vi "GUI_CH1_Comm_ZEROMQ.vi"() -> ()   [LabVIEW 2018]
uses:
  RxTx/RxTx.lvclass
  <vilib>/addons/zeromq/socket_type.ctl
  <vilib>/addons/zeromq/zmq_context.lvclass
  <vilib>/addons/zeromq/zeromq.lvlib
  <vilib>/addons/zeromq/zmq_socket.lvclass
panel:
  out "error out 4":errorcluster
  out "error out":errorcluster
  in  "IP":string="200.131.64.49"
  in  "stop":bool
  out "error out 3":errorcluster
  out "error out 2":errorcluster
  in  "RxTx.lvclass 2":refnum<class "RxTx.lvclass">
  in  "Channel":u16=1
  # "Channel 1 - TCPIP Communication"
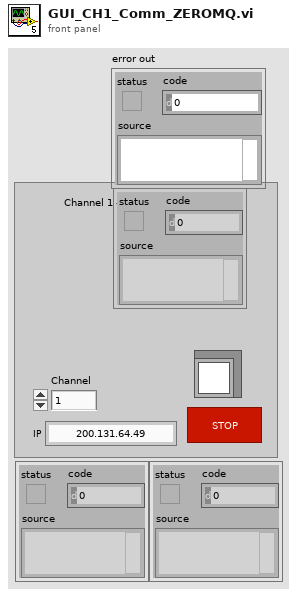
[diagram p1: front panel]
types:
  T1 = typedef "zeromq.lvlib/socket_type.ctl" = enum8{"ZMQ_PAIR", "ZMQ_PUB", "ZMQ_SUB", "ZMQ_REQ", "ZMQ_REP", "ZMQ_DEALER", "ZMQ_ROUTER", "ZMQ_PULL", "ZMQ_PUSH", "ZMQ_XPUB", "ZMQ_XSUB", "ZMQ_STREAM", "ZMQ_SERVER", "ZMQ_CLIENT", "ZMQ_RADIO", "ZMQ_DISH", "ZMQ_GATHER", "ZMQ_SCATTER", "ZMQ_DGRAM"}
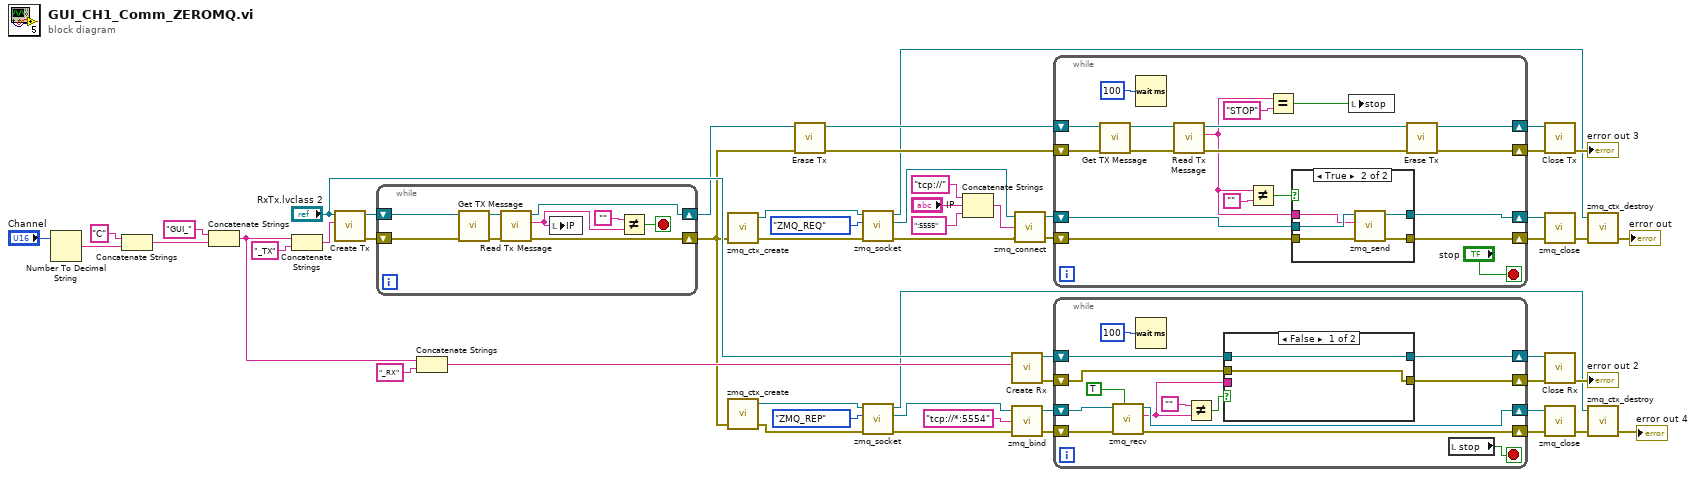
[diagram p0: block diagram]
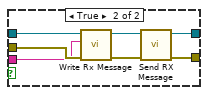
[diagram p3: hidden frame]
diagram:
  n1 = Number To Decimal String(number="Channel") -> (decimal integer string=w51:string)  [unwired: 1 in]
  n2 = Concatenate Strings("C", w51) -> (w36:string)
  n3 = Concatenate Strings("GUI_", w36) -> (w37:string)
  n4 = Concatenate Strings(w37, "_TX" ("Reader Name")) -> (w45:string)
  n5 = call "Create Tx.vi"("Writer Name"=w45, "RxTx in"="RxTx.lvclass 2") -> ("error out"=w31:errorcluster, "RxTx out"=w32:refnum<class "RxTx.lvclass">)  [unwired: 8 in]
  n6 = while {
    shift-right: [w59] -> w14
    shift-left: w31 -> [w58]
    shift-right: [w57] -> w35
    shift-left: w32 -> [w56]
    stop <- w60 stop-if-true
    n7 = call "Get TX Message.vi"("error in (no error)"=w58, "RxTx in"=w56) -> ("error out"=w62:errorcluster, "RxTx out"=w63:refnum<class "RxTx.lvclass">)  [unwired: 8 in]
    n8 = call "Read Tx Message.vi"("error in (no error)"=w62, "RxTx in"=w63) -> ("error out"=w59:errorcluster, "Tx Message"=w55:string, "RxTx out"=w57:refnum<class "RxTx.lvclass">)  [unwired: 7 in]
    n9 = local write "IP"(w55) -> ()
    n10 = Not Equal?(x="", y=w55) -> (x != y?=w60:bool)
  }
  n11 = Concatenate Strings(w37, "_RX" ("Reader Name")) -> (w54:string)
  n12 = call <vilib>:"zmq_ctx_create.vi"("error in"=w14) -> ("error out"=w20:errorcluster, "context out"=w21:refnum<class "zmq_context.lvclass">)  [unwired: 3 in]
  n13 = call <vilib>:"zmq_ctx_create.vi"("error in"=w14) -> ("error out"=w28:errorcluster, "context out"=w29:refnum<class "zmq_context.lvclass">)  [unwired: 3 in]
  n14 = call "Erase Tx.vi"("error in (no error)"=w14, "RxTx in"=w35) -> ("error out"=w33:errorcluster, "RxTx out"=w34:refnum<class "RxTx.lvclass">)  [unwired: 8 in]
  n15 = call <vilib>:"zmq_socket.vi"("error in"=w20, "socket type"=socket_type."ZMQ_REQ", "context in"=w21) -> ("error out"=w2:errorcluster, "socket out"=w4:refnum<class "zmq_socket.lvclass">, "context out"=w13:refnum<class "zmq_context.lvclass">)  [unwired: 2 in]
  n16 = call <vilib>:"zmq_socket.vi"("error in"=w28, "socket type"=socket_type."ZMQ_REP", "context in"=w29) -> ("error out"=w11:errorcluster, "socket out"=w12:refnum<class "zmq_socket.lvclass">, "context out"=w24:refnum<class "zmq_context.lvclass">)  [unwired: 2 in]
  n17 = Concatenate Strings("tcp://" ("endpoint"), "IP", ":5555" ("endpoint")) -> (w3:string)
  n18 = call "Create Rx.vi"("Reader Name"=w54, "RxTx in"="RxTx.lvclass 2") -> ("error out"=w49:errorcluster, "RxTx out"=w50:refnum<class "RxTx.lvclass">)  [unwired: 8 in]
  n19 = call <vilib>:"zmq_bind.vi"("error in"=w11, "endpoint"="tcp://*:5554", "socket in"=w12) -> ("error out"=w10:errorcluster, "socket out"=w9:refnum<class "zmq_socket.lvclass">)  [unwired: 1 in]
  n20 = call <vilib>:"zmq_connect.vi"("error in"=w2, "endpoint"=w3, "socket in"=w4) -> ("error out"=w6:errorcluster, "socket out"=w5:refnum<class "zmq_socket.lvclass">)  [unwired: 1 in]
  n21 = while {
    shift-right: [w82] -> w43
    shift-left: w34 -> [w75]
    shift-right: [w81] -> w42
    shift-left: w33 -> [w74]
    shift-right: [w69] -> w17
    shift-left: w6 -> [w70]
    shift-right: [w68] -> w16
    shift-left: w5 -> [w71]
    stop <- "stop" stop-if-true
    n22 = call "Get TX Message.vi"("error in (no error)"=w74, "RxTx in"=w75) -> ("error out"=w80:errorcluster, "RxTx out"=w76:refnum<class "RxTx.lvclass">)  [unwired: 8 in]
    n23 = Wait (ms)(milliseconds to wait=u32 100) -> ()  [unwired: 1 out]
    n24 = call "Read Tx Message.vi"("error in (no error)"=w80, "RxTx in"=w76) -> ("error out"=w77:errorcluster, "Tx Message"=w67:string, "RxTx out"=w78:refnum<class "RxTx.lvclass">)  [unwired: 7 in]
    n25 = Not Equal?(x=w67, y="") -> (x != y?=w64:bool)
    n26 = Equal?(x=w67, y="STOP" ("endpoint")) -> (x = y?=w65:bool)
    n27 = case shown="True" w64 {
      tunnel: w67 -> [_ w85]
      tunnel: w71 -> [w84 w89]
      tunnel: w70 -> [w83 w88]
      tunnel: [w83 w87] -> w69
      tunnel: [w84 w86] -> w68
      frame False {
      }
      frame True {
        n28 = call <vilib>:"zmq_send.vi"("error in"=w88, "data"=w85, "socket in"=w89) -> ("error out"=w87:errorcluster, "socket out"=w86:refnum<class "zmq_socket.lvclass">)  [unwired: 4 in]
      }
    }
    n29 = local write "stop"(w65) -> ()
    n30 = call "Erase Tx.vi"("error in (no error)"=w77, "RxTx in"=w78) -> ("error out"=w81:errorcluster, "RxTx out"=w82:refnum<class "RxTx.lvclass">)  [unwired: 8 in]
  }
  n31 = while {
    shift-right: [w98] -> w47
    shift-left: w49 -> [w103]
    shift-right: [w99] -> w48
    shift-left: w50 -> [w102]
    shift-right: [w96] -> w26
    shift-left: w9 -> [w90]
    shift-right: [w95] -> w25
    shift-left: w10 -> [w91]
    stop <- w97 stop-if-true
    n32 = call <vilib>:"zmq_recv.vi"("no block? (F)"=TRUE, "error in"=w91, "socket in"=w90) -> ("error out"=w95:errorcluster, "data"=w94:string, "socket out"=w96:refnum<class "zmq_socket.lvclass">)  [unwired: 2 in, 2 out]
    n33 = Wait (ms)(milliseconds to wait=u32 100) -> ()  [unwired: 1 out]
    n34 = Not Equal?(x="", y=w94) -> (x != y?=w100:bool)
    n35 = case shown="False" w100 {
      tunnel: w103 -> [w104 w110]
      tunnel: w102 -> [w105 w109]
      tunnel: [w105 w108] -> w99
      tunnel: [w104 w107] -> w98
      tunnel: w94 -> [_ w106]
      frame False {
      }
      frame True {
        n36 = call "Write Rx Message.vi"("error in (no error)"=w110, "Rx Message"=w106, "RxTx in"=w109) -> ("error out"=w111:errorcluster, "RxTx out"=w112:refnum<class "RxTx.lvclass">)  [unwired: 7 in]
        n37 = call "Send RX Message.vi"("error in (no error)"=w111, "RxTx in"=w112) -> ("error out"=w107:errorcluster, "RxTx out"=w108:refnum<class "RxTx.lvclass">)  [unwired: 8 in]
      }
    }
    n38 = local read "stop"() -> (w97:bool)
  }
  n39 = call "Close Tx.vi"("error in (no error)"=w42, "RxTx in"=w43) -> ("error out"=→"error out 3":errorcluster)  [unwired: 8 in, 1 out]
  n40 = call <vilib>:"zmq_close.vi"("error in"=w17, "socket"=w16) -> ("error out"=w18:errorcluster)  [unwired: 3 in]
  n41 = call "Close Rx.vi"("error in (no error)"=w47, "RxTx in"=w48) -> ("error out"=→"error out 2":errorcluster)  [unwired: 8 in, 1 out]
  n42 = call <vilib>:"zmq_close.vi"("error in"=w25, "socket"=w26) -> ("error out"=w27:errorcluster)  [unwired: 3 in]
  n43 = call <vilib>:"zmq_ctx_destroy.vi"("error in"=w18, "context in"=w13) -> ("error out"=→"error out":errorcluster)  [unwired: 3 in]
  n44 = call <vilib>:"zmq_ctx_destroy.vi"("error in"=w27, "context in"=w24) -> ("error out"=→"error out 4":errorcluster)  [unwired: 3 in]
